vi "Set-deposition.vi"(8 "error in (no error)":errorcluster, 10 "Depositing?":bool, 11 "Object ref in":T1) -> (0 "error out":errorcluster, 3 "Object ref out":T1)   [LabVIEW 2013, in "SLMControl.lvlib" / "SC-Main.lvclass"]
uses:
  SC-Main.lvclass
  Object-reference.ctl
  UI/Control-names.ctl
  SC-Main.lvclass/SC-Main.ctl
  Read Deposition notif.vi
  Read UI.vi
  UI/SC-UI.lvclass
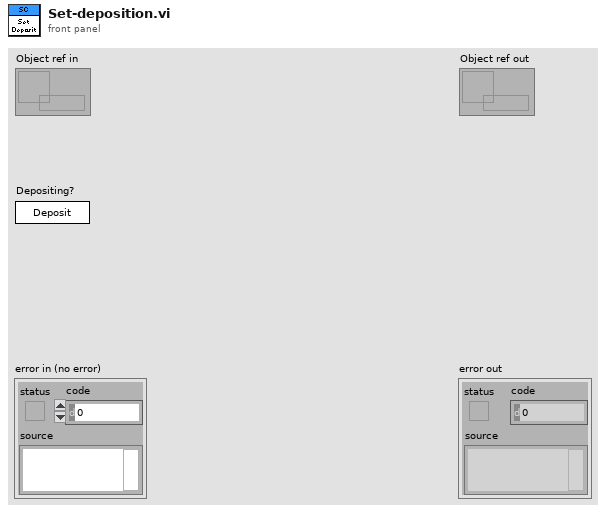
[diagram p1: front panel]
types:
  T1 = typedef "SLMControl.lvlib/SC-Main.lvclass/Object-reference.ctl" = refnum<data-value>
  T2 = typedef "SLMControl.lvlib/SC-UI.lvclass/Control-names.ctl" = enum16{"Com-in", "Com-out", "Help", "Status", "Load configuration", "Save configuration", "Load lasing files", "Load deposition files", "Clear", "Files", "Activate", "Execute", "Abort", "Options", "Current layer", "Current iteration", "Last elapsed time", "Deposition status", "Lasing job", "Status LEDs", "Exiting led", "Initialized led", "Files loaded led", "Activated led", "Executing led", "Deposition led", "Lasing job led", "Lasing led"}
  T3 = typedef "SLMControl.lvlib/SC-UI.lvclass/Panes-reference.ctl" = refnum<data-value>
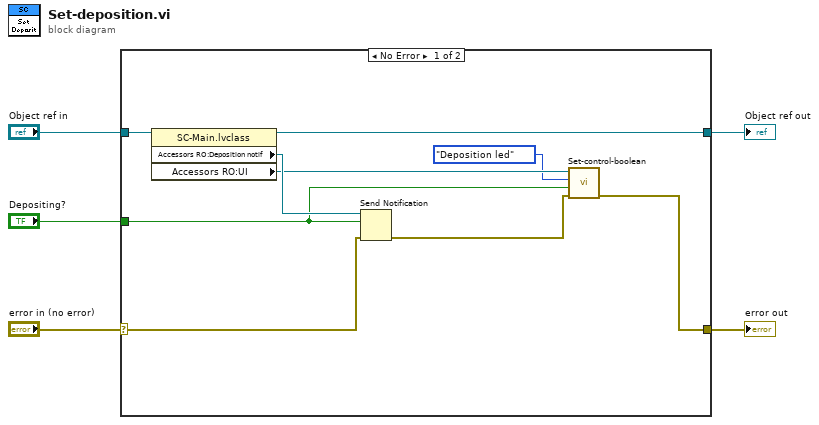
[diagram p0: block diagram]
diagram:
  n1 = case shown="No Error" "error in (no error)" {
    selector: "error in (no error)" -> [w11 w16]
    tunnel: [w8 w16] -> w4
    tunnel: [w13 w15] -> w2
    tunnel: "Object ref in" -> [w14 w15]
    tunnel: "Depositing?" -> [w6 _]
    frame No Error {
      n2 = property class="SC-Main.lvclass"(reference=w14) -> (reference out=w13:T1, "Accessors RO:Deposition notif"=w12:refnum<notifier>, "Accessors RO:UI"=w10:T3)  [unwired: 1 in, 1 out]
      n3 = Send Notification(notification=w6, notifier=w12, error in (no error)=w11) -> (error out=w9:errorcluster)  [unwired: 1 out]
      n4 = call "Set-control-boolean.vi"("error in (no error)"=w9, "Value"=w6, "Control name"=Control-names."Deposition led", "Panes in"=w10) -> ("error out"=w8:errorcluster)  [unwired: 6 in, 1 out]
    }
    frame Error {
    }
  }
  "error out" <- w4
  "Object ref out" <- w2
